vi "Write Position.vi"(8 "Error In":errorcluster, 10 "Position":u64, 11 "SFTP File In":refnum<class "SFTP File.lvclass">) -> (0 "Error Out":errorcluster, 3 "SFTP File Out":refnum<class "SFTP File.lvclass">)   [LabVIEW 2018, in "Toolkit.lvlib" / "SFTP File.lvclass"]
uses:
  SFTP File.lvclass
  SFTP File.lvclass/SFTP File.ctl
  SFTP/SFTP.lvclass/SFTP.ctl
  Toolkit.lvlib
  SFTP/SFTP.lvclass
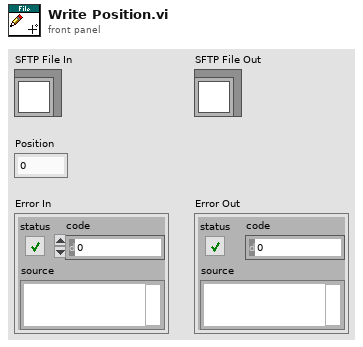
[diagram p1: front panel]
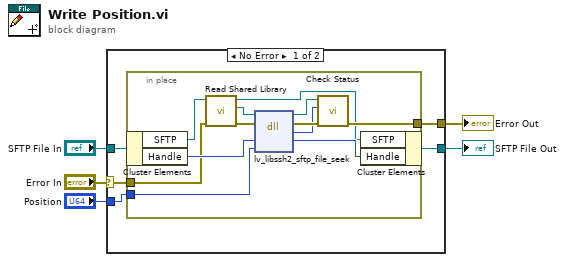
[diagram p0: block diagram]
diagram:
  n1 = case shown="No Error" "Error In" {
    selector: "Error In" -> [w9 w23]
    tunnel: "SFTP File In" -> [w10 w24]
    tunnel: [w8 w24] -> w2
    tunnel: [w7 w23] -> w3
    tunnel: "Position" -> [w6 _]
    frame No Error {
      n2 = in-place {
        in-place-border: w9 -> [w21]
        in-place-border: [w16] -> w7
        in-place-border: w6 -> [w11]
        n3 = in-place-cluster #1(w10) -> ("SFTP"=w14:refnum<class "SFTP.lvclass">, "Handle"=w22:u64)
        n4 = call "Read Shared Library.vi"("Error In"=w21, "SFTP In"=w14) -> ("Erorr Out"=w15:errorcluster, "lv-libssh2 Shared Library"=w12:path, "SFTP Out"=w13:refnum<class "SFTP.lvclass">)  [unwired: 7 in]
        n5 = dll-call lib="libssh2lv.*" fn="lv_libssh2_sftp_file_seek"(path in=w12, error in=w15, "handle"=w22, "offset"=w11) -> (path out=w18:path, error out=w19:errorcluster, "status"=w17:i32, "handle"=w20:u64)  [unwired: 2 in]
        n6 = call "Check Status.vi"("Error In"=w19, "Status"=w17, "lv-libssh2 Shared Library In"=w18) -> ("Error Out"=w16:errorcluster)  [unwired: 7 in, 1 out]
        n7 = in-place-cluster #1("SFTP"=w13, "Handle"=w20) -> (w8:refnum<class "SFTP File.lvclass">)
      }
    }
    frame Error {
    }
  }
  "Error Out" <- w3
  "SFTP File Out" <- w2
